vi "sequence structure read.vi"   [LabVIEW 2015]
uses:
  <vilib>/Platform/TimedLoop/XDataNode/timing_clust.ctl
  <vilib>/Platform/TimedLoop/XDataNode/nitl_modes.ctl
  <vilib>/Platform/TimedLoop/XDataNode/wakeup.ctl
  Robot Global Data.vi
  <vilib>/platform/TimedLoop/XDataNode/XDataNode.xnode
  <vilib>/Platform/TimedLoop/XDataNode/XDNodeRunTimeDep.lvlib
types:
  T1 = typedef "WPI_MotorControlDeviceRef.ctl" = cluster{"DeviceStatus":errorcluster, "Type":T2, "PWM":cluster{"PWM Channel":T3, "DeadBand":T4}, "CAN":cluster{"Device Number":u8, "Control Mode":T5, "Semaphore":T6, "Max Vout":dbl, "TalonSRX Control Mode":T7}, "Invert":bool}
  T2 = typedef "WPI_MotorControlType.ctl" = enum16{"PWM", "CAN", "CANTalonSRX"}
  T3 = typedef "FPGA_DIOPWMChannel.ctl" = enum8{"PWM 0", "PWM 1", "PWM 2", "PWM 3", "PWM 4", "PWM 5", "PWM 6", "PWM 7", "PWM 8", "PWM 9", "PWM MXP 0", "PWM MXP 1", "PWM MXP 2", "PWM MXP 3", "PWM MXP 4", "PWM MXP 5", "PWM MXP 6", "PWM MXP 7", "PWM MXP 8", "PWM MXP 9", "Invalid"}
  T4 = typedef "WPI_PWMDeadband.ctl" = cluster{"Name":string, "maxPositivePwm":i32, "minPositivePwm":i32, "centerPwm":i32, "maxNegativePwm":i32, "minNegativePwm":i32, "angularRange":u16}
  T5 = typedef "WPI_CANJaguar_ControlMode.ctl" = enum8{"Percent VBus", "Current", "Speed", "Position", "Voltage"}
  T6 = typedef "Semaphore RefNum" = refnum<k1>
  T7 = typedef "WPI_CANTalonSRX_APIControlMode.ctl" = enum8{"Percent VBus", "Speed", "Position", "Slave", "Unchanged / Invalid", "Voltage Compensation", "Current", "Motion Profile"}
  T8 = enum16{"open", "open or create", "create or replace", "create", "open (read-only)"}
  T9 = typedef "XDNodeRunTimeDep.lvlib/timing_clust.ctl" = cluster{"Expected End [f-1]":u64, "Actual End [f-1]":u64, "Finished Late? [f-1]":bool, "Expected End [i-1]":u64, "Actual End [i-1]":u64, "Finished Late? [i-1]":bool, "Expected Start [i]":u64, "Actual Start [i]":u64, "Expected Start [f]":u64, "Actual Start [f]":u64, "Source Name":string, "Structure Name":string, "Period":i64, "Deadline":i64, "Offset":i64, "Start":i64, "Priority":i32, "Timeout":i32, "Mode":T10, "Wakeup Reason":T11, "Error":errorcluster, "Source Type":string, "Secondary Source Type":string, "Global End Time":u64, "Global Start Time":u64, "Frame Duration":u64, "Iteration Duration":u64, "Assigned CPU":i32, "I/O Scan Engine Mode":u32}
  T10 = typedef "XDNodeRunTimeDep.lvlib/nitl_modes.ctl" = enum32{"No Change", "Process missed periods, maintain original phase", "Discard missed periods, maintain original phase", "Process missed periods, ignore original phase", "Discard missed periods, ignore original phase"}
  T11 = typedef "XDNodeRunTimeDep.lvlib/wakeup.ctl" = enum32{"Normal", "Aborted", "Asynchronous wakeup", "Timing source error", "Timed loop error", "Timeout"}
  T12 = enum16{"open", "replace", "create", "open or create", "replace or create", "replace or create with confirmation"}
  T13 = cluster{"Record?":bool, "Current File":string, "Run script?":bool, "Stop recording?":bool, "Stop script?":bool}
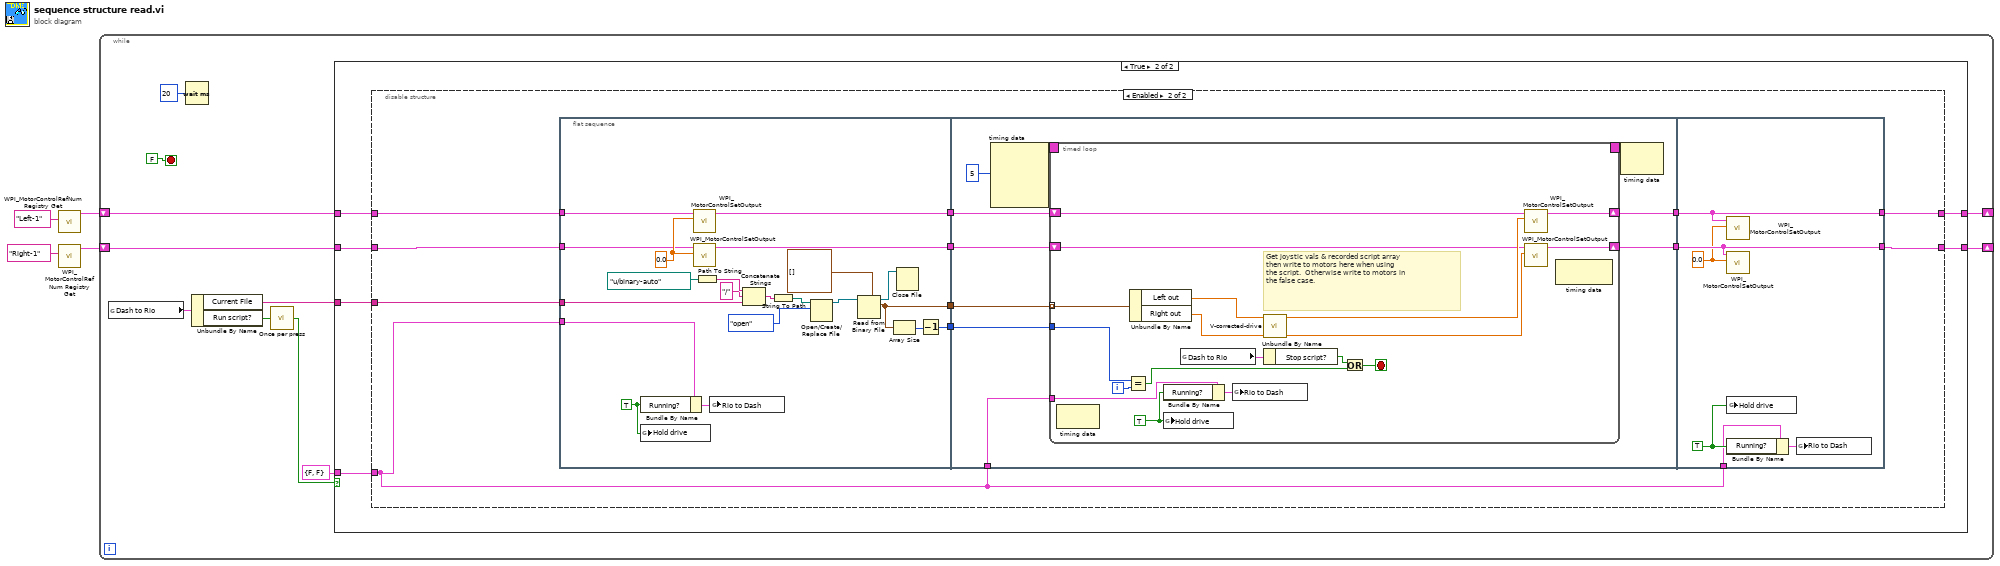
[diagram p0: block diagram]
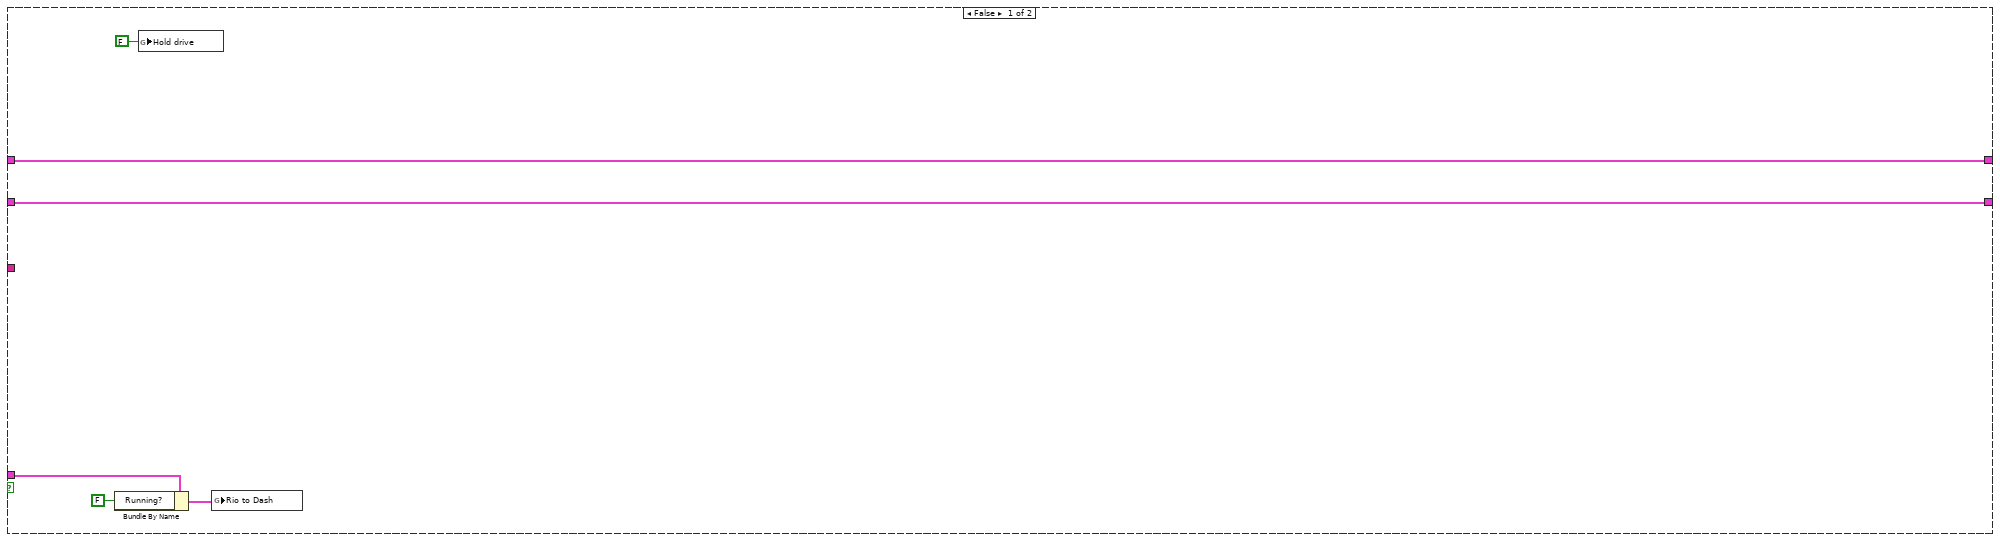
[diagram p2: hidden frame]
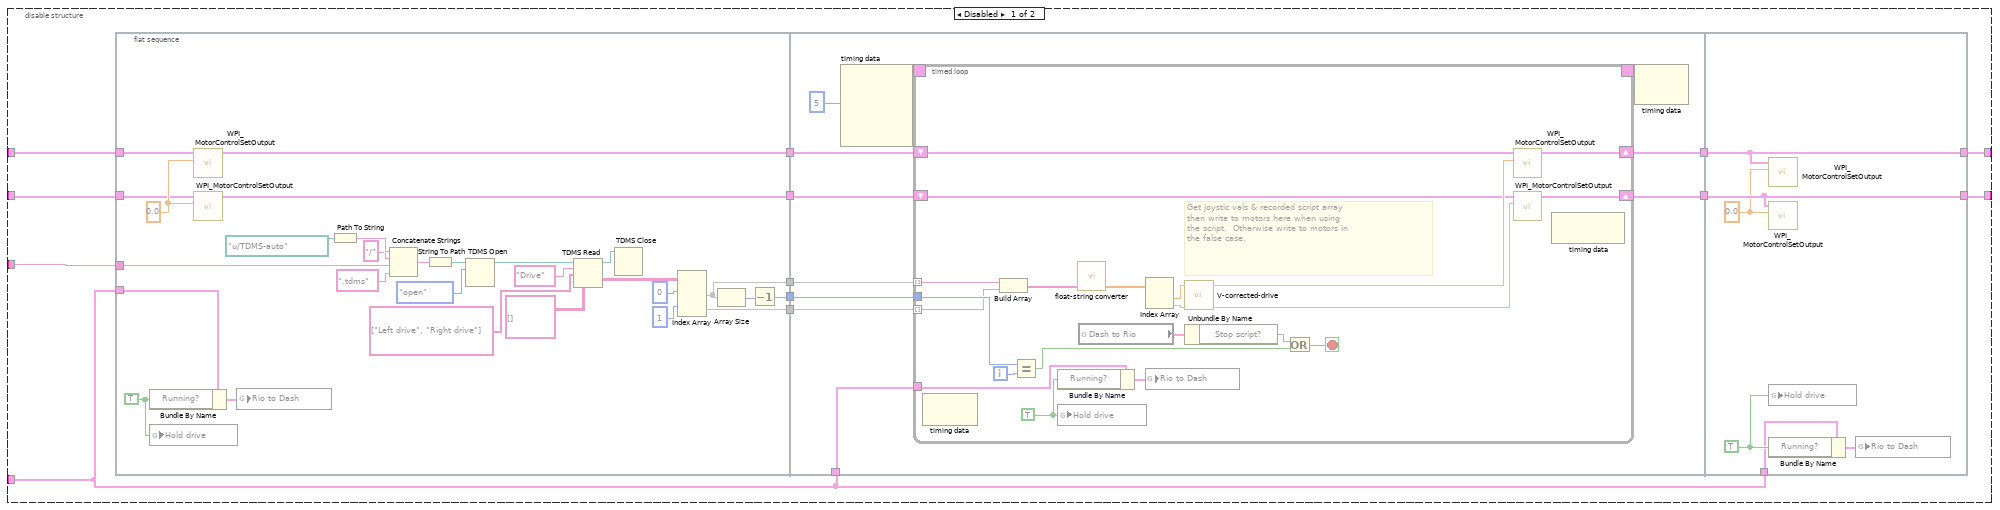
[diagram p3: hidden frame]
diagram:
  n1 = call <vilib>:"WPI_MotorControlRefNum Registry Get.vi"("refnum name"="Left-1") -> ("MotorControlDevRef"=w1:T1)  [unwired: 9 in, 1 out]
  n2 = call <vilib>:"WPI_MotorControlRefNum Registry Get.vi"("refnum name"="Right-1") -> ("MotorControlDevRef"=w2:T1)  [unwired: 9 in, 1 out]
  n3 = while {
    shift-right: [w12] -> _
    shift-left: w2 -> [w11]
    shift-right: [w10] -> _
    shift-left: w1 -> [w13]
    stop <- FALSE stop-if-true
    n4 = global read "Robot Global Data.vi" "Dash to Rio"() -> (w7:T13)
    n5 = Wait (ms)(milliseconds to wait=u32 20) -> ()  [unwired: 1 out]
    n6 = Unbundle By Name(w7) -> ("Current File"=w6:string, "Run script?"=w8:bool)
    n7 = call "Once per press.vi"("In"=w8) -> ("Out"=w9:bool)  [unwired: 2 in]
    n8 = case shown="True" w9 {
      tunnel: w13 -> [w21 w27]
      tunnel: w11 -> [w20 w26]
      tunnel: [w21 w25] -> w10
      tunnel: [w20 w24] -> w12
      tunnel: w6 -> [_ w23]
      tunnel: cluster{"Recording?":bool, "Running?":bool} {"Recording?"=FALSE, "Running?"=FALSE} ("Rio to Dash") -> [w17 w22]
      frame False {
        n9 = Bundle By Name(cluster=w17, "Running?"=FALSE) -> (w18:cluster{"Recording?":bool, "Running?":bool})
        n10 = global write "Robot Global Data.vi" "Hold drive"(FALSE) -> ()
        n11 = global write "Robot Global Data.vi" "Rio to Dash"(w18) -> ()
      }
      frame True {
        n12 = disable-structure shown="Enabled" {
          disable-tunnel: w27 -> [w33 w119]
          disable-tunnel: w26 -> [w32 w118]
          disable-tunnel: [w31 w114] -> w25
          disable-tunnel: [w30 w113] -> w24
          disable-tunnel: w23 -> [w29 w117]
          disable-tunnel: w22 -> [w28 w115]
          frame Disabled {
            n13 = flat-sequence {
              tunnel: [w62] -> w40
              tunnel: [w60] -> w39
              tunnel: [w64] -> w38
              tunnel: [w58] -> w37
              tunnel: [w57] -> w36
              tunnel: w33 -> [w55]
              tunnel: w32 -> [w54]
              tunnel: w29 -> [w45]
              tunnel: w28 -> [w42]
              tunnel: w40 -> [w77]
              tunnel: w39 -> [w79]
              tunnel: w38 -> [w78]
              tunnel: w37 -> [w73]
              tunnel: w36 -> [w72]
              tunnel: [w71] -> w35
              tunnel: [w70] -> w34
              tunnel: w28 -> [w69]
              tunnel: w35 -> [w112]
              tunnel: w34 -> [w111]
              tunnel: [w112] -> w31
              tunnel: [w111] -> w30
              tunnel: w28 -> [w107]
              frame #0 {
                w41 = TRUE
                w56 = 0.0
                n14 = Bundle By Name(cluster=w42, "Running?"=w41) -> (w43:cluster{"Recording?":bool, "Running?":bool})
                n15 = global write "Robot Global Data.vi" "Hold drive"(w41) -> ()
                n16 = call <vilib>:"WPI_MotorControlSetOutput.vi"("Output"=w56, "MotorControlDevRef"=w55) -> ("MotorControlDevRef"=w58:T1)  [unwired: 7 in, 2 out]
                n17 = call <vilib>:"WPI_MotorControlSetOutput.vi"("Output"=w56, "MotorControlDevRef"=w54) -> ("MotorControlDevRef"=w57:T1)  [unwired: 7 in, 2 out]
                n18 = global write "Robot Global Data.vi" "Rio to Dash"(w43) -> ()
                n19 = Path To String(path=path "u:/TDMS-auto" ("file path 3")) -> (string=w50:string)
                n20 = Concatenate Strings(w50, "/" ("string"), w45, ".tdms" ("string")) -> (w49:string)
                n21 = String To Path(string=w49) -> (path=w52:path)
                n22 = TDMS Open(10:T8."open" ("operation (0:open)"), 11:w52) -> (3:w46:refnum<k34>)  [unwired: 5 in, 1 out]
                n23 = TDMS Read(0:w46, 5:"Drive" ("group name in"), 7:string[] ["Left drive", "Right drive"] ("channel name(s) in"), 12:string[][] [] ("array w/ subset deleted")) -> (4:w44:refnum<k34>, 10:w65:string[][])  [unwired: 4 in, 4 out]
                n24 = TDMS Close(11:w44) -> ()  [unwired: 1 in, 2 out]
                n25 = Index Array(array=w65, index (row) #1=0, index (row) #2=1 ("index (row)")) -> (element #1=w60:string[], element #2=w64:string[])  [unwired: 2 in]
                n26 = Array Size(array=w60) -> (size(s)=w59:i32)
                n27 = Decrement(x=w59) -> (x-1=w62:i32)
              }
              frame #1 {
                n28 = node-c288(i64 5 ("Period")) -> (w76:T9)  [unwired: 3 in]
                n29 = timed-loop {
                  tunnel: w79 -> [w95] mode=indexing
                  tunnel: w78 -> [w96] mode=indexing
                  tunnel: w77 -> [w99]
                  timing: w76 -> [_]
                  timing-out: [_] -> w75
                  shift-right: [w86] -> w71
                  shift-left: w73 -> [w88]
                  shift-right: [w85] -> w70
                  shift-left: w72 -> [w87]
                  tunnel: w69 -> [w80]
                  i -> [w100]
                  stop <- w98 stop-if-true
                  w81 = TRUE
                  # "Get joystic vals & recorded script array\nthen write to motors here when using\nthe script.  Otherwise write to motors in \nthe false case."
                  n30 = node-c288() -> ()  [unwired: 1 in, 1 out]
                  n31 = Build Array(w95, w96) -> (w94:string[])
                  n32 = Equal?(x=w99, y=w100) -> (x = y?=w97:bool)
                  n33 = Bundle By Name(cluster=w80, "Running?"=w81) -> (w82:cluster{"Recording?":bool, "Running?":bool})
                  n34 = global write "Robot Global Data.vi" "Hold drive"(w81) -> ()
                  n35 = call "float-string converter.vi"("float string in"=w94) -> ("float out"=w93:dbl[])  [unwired: 3 in, 1 out]
                  n36 = global read "Robot Global Data.vi" "Dash to Rio"() -> (w84:T13)
                  n37 = Index Array(array=w93) -> (element #1=w90:dbl, element #2=w89:dbl)  [unwired: 2 in]
                  n38 = global write "Robot Global Data.vi" "Rio to Dash"(w82) -> ()
                  n39 = call "V-corrected-drive.vi"("R-IN"=w89, "L-IN 2"=w90) -> ("Right out"=w92:dbl, "Left out"=w91:dbl)  [unwired: 8 in]
                  n40 = Unbundle By Name(w84) -> ("Stop script?"=w83:bool)
                  n41 = Or(x=w83, y=w97) -> (x .or. y?=w98:bool)
                  n42 = call <vilib>:"WPI_MotorControlSetOutput.vi"("Output"=w91, "MotorControlDevRef"=w88) -> ("MotorControlDevRef"=w86:T1)  [unwired: 7 in, 2 out]
                  n43 = call <vilib>:"WPI_MotorControlSetOutput.vi"("Output"=w92, "MotorControlDevRef"=w87) -> ("MotorControlDevRef"=w85:T1)  [unwired: 7 in, 2 out]
                  n44 = node-c288() -> ()  [unwired: 1 in, 1 out]
                }
                n45 = node-c288(w75) -> ()  [unwired: 1 out]
              }
              frame #2 {
                w108 = TRUE
                w110 = 0.0
                n46 = call <vilib>:"WPI_MotorControlSetOutput.vi"("Output"=w110, "MotorControlDevRef"=w112) -> ()  [unwired: 7 in, 3 out]
                n47 = call <vilib>:"WPI_MotorControlSetOutput.vi"("Output"=w110, "MotorControlDevRef"=w111) -> ()  [unwired: 7 in, 3 out]
                n48 = global write "Robot Global Data.vi" "Hold drive"(w108) -> ()
                n49 = Bundle By Name(cluster=w107, "Running?"=w108) -> (w109:cluster{"Recording?":bool, "Running?":bool})
                n50 = global write "Robot Global Data.vi" "Rio to Dash"(w109) -> ()
              }
            }
          }
          frame Enabled {
            n51 = flat-sequence {
              tunnel: [w145] -> w124
              tunnel: [w143] -> w123
              tunnel: [w142] -> w122
              tunnel: w119 -> [w140]
              tunnel: w118 -> [w139]
              tunnel: w117 -> [w134]
              tunnel: w115 -> [w132]
              tunnel: [w125] -> w116
              tunnel: w124 -> [w155]
              tunnel: w123 -> [w151]
              tunnel: w122 -> [w150]
              tunnel: [w149] -> w121
              tunnel: [w148] -> w120
              tunnel: w115 -> [w147]
              tunnel: w116 -> [w146]
              tunnel: w121 -> [w185]
              tunnel: w120 -> [w184]
              tunnel: [w185] -> w114
              tunnel: [w184] -> w113
              tunnel: w115 -> [w180]
              frame #0 {
                w131 = TRUE
                w141 = 0.0
                n52 = Bundle By Name(cluster=w132, "Running?"=w131) -> (w133:cluster{"Recording?":bool, "Running?":bool})
                n53 = global write "Robot Global Data.vi" "Hold drive"(w131) -> ()
                n54 = call <vilib>:"WPI_MotorControlSetOutput.vi"("Output"=w141, "MotorControlDevRef"=w140) -> ("MotorControlDevRef"=w143:T1)  [unwired: 7 in, 2 out]
                n55 = call <vilib>:"WPI_MotorControlSetOutput.vi"("Output"=w141, "MotorControlDevRef"=w139) -> ("MotorControlDevRef"=w142:T1)  [unwired: 7 in, 2 out]
                n56 = Path To String(path=path "u:/binary-auto" ("file path 3")) -> (string=w137:string)
                n57 = global write "Robot Global Data.vi" "Rio to Dash"(w133) -> ()
                n58 = Concatenate Strings(w137, "/" ("string"), w134) -> (w136:string)
                n59 = String To Path(string=w136) -> (path=w129:path)
                n60 = Open/Create/Replace File(file path (use dialog)=w129, operation (0:open)=T12."open") -> (refnum out=w128:refnum<file>)  [unwired: 4 in, 2 out]
                n61 = Read from Binary File(5:cluster{"Left out":dbl, "Right out":dbl}[] [], 11:w128) -> (2:w125:cluster{"Left out":dbl, "Right out":dbl}[], 3:w126:refnum<file>)  [unwired: 4 in, 2 out]
                n62 = Array Size(array=w125) -> (size(s)=w144:i32)
                n63 = Close File(refnum=w126) -> ()  [unwired: 1 in, 2 out]
                n64 = Decrement(x=w144) -> (x-1=w145:i32)
              }
              frame #1 {
                n65 = node-c288(i64 5 ("Period")) -> (w154:T9)  [unwired: 3 in]
                n66 = timed-loop {
                  tunnel: w155 -> [w172]
                  timing: w154 -> [_]
                  timing-out: [_] -> w153
                  shift-right: [w165] -> w149
                  shift-left: w151 -> [w167]
                  shift-right: [w164] -> w148
                  shift-left: w150 -> [w166]
                  tunnel: w147 -> [w159]
                  tunnel: w146 -> [w158] mode=indexing
                  i -> [w173]
                  stop <- w171 stop-if-true
                  w160 = TRUE
                  # "Get joystic vals & recorded script array\nthen write to motors here when using\nthe script.  Otherwise write to motors in \nthe false case."
                  n67 = node-c288() -> ()  [unwired: 1 in, 1 out]
                  n68 = Equal?(x=w172, y=w173) -> (x = y?=w170:bool)
                  n69 = Unbundle By Name(w158) -> ("Left out"=w157:dbl, "Right out"=w156:dbl)
                  n70 = Bundle By Name(cluster=w159, "Running?"=w160) -> (w161:cluster{"Recording?":bool, "Running?":bool})
                  n71 = global write "Robot Global Data.vi" "Hold drive"(w160) -> ()
                  n72 = global read "Robot Global Data.vi" "Dash to Rio"() -> (w163:T13)
                  n73 = global write "Robot Global Data.vi" "Rio to Dash"(w161) -> ()
                  n74 = call "V-corrected-drive.vi"("R-IN"=w156, "L-IN 2"=w157) -> ("Right out"=w169:dbl, "Left out"=w168:dbl)  [unwired: 8 in]
                  n75 = Unbundle By Name(w163) -> ("Stop script?"=w162:bool)
                  n76 = Or(x=w162, y=w170) -> (x .or. y?=w171:bool)
                  n77 = call <vilib>:"WPI_MotorControlSetOutput.vi"("Output"=w168, "MotorControlDevRef"=w167) -> ("MotorControlDevRef"=w165:T1)  [unwired: 7 in, 2 out]
                  n78 = call <vilib>:"WPI_MotorControlSetOutput.vi"("Output"=w169, "MotorControlDevRef"=w166) -> ("MotorControlDevRef"=w164:T1)  [unwired: 7 in, 2 out]
                  n79 = node-c288() -> ()  [unwired: 1 in, 1 out]
                }
                n80 = node-c288(w153) -> ()  [unwired: 1 out]
              }
              frame #2 {
                w181 = TRUE
                w183 = 0.0
                n81 = call <vilib>:"WPI_MotorControlSetOutput.vi"("Output"=w183, "MotorControlDevRef"=w185) -> ()  [unwired: 7 in, 3 out]
                n82 = call <vilib>:"WPI_MotorControlSetOutput.vi"("Output"=w183, "MotorControlDevRef"=w184) -> ()  [unwired: 7 in, 3 out]
                n83 = global write "Robot Global Data.vi" "Hold drive"(w181) -> ()
                n84 = Bundle By Name(cluster=w180, "Running?"=w181) -> (w182:cluster{"Recording?":bool, "Running?":bool})
                n85 = global write "Robot Global Data.vi" "Rio to Dash"(w182) -> ()
              }
            }
          }
        }
      }
    }
  }
